vi "Begin.vi"() -> (1 "CameraDevRef":T1)   [LabVIEW 2011]
doc: "Called before other user functions, this VI is expected to open initial I/O refnums, load in file data, and do all program initialization. Notice that the <B>error out</B> terminal is simply used for data flow. Wiring it to other structures or subVIs ensures that this VI runs first."
uses:
  <vilib>/Rock Robotics/WPI/Camera/WPI_CameraDevRef.ctl
  <vilib>/Rock Robotics/SystemInterfaces/DIO/FPGA_DIOPWMChannel.ctl
  <vilib>/Rock Robotics/WPI/Joystick/WPI_JoystickDeviceEnum.ctl
  <vilib>/Rock Robotics/SystemInterfaces/AI/FPGA_AIChannel.ctl
  <vilib>/Rock Robotics/SystemInterfaces/DIO/FPGA_DIORelayChannel.ctl
  <vilib>/Rock Robotics/SystemInterfaces/DIO/FPGA_DIOChannel.ctl
  <vilib>/Rock Robotics/SystemInterfaces/AI/FPGA_AIGyroChannel.ctl
  <vilib>/Rock Robotics/WPI/Relay/WPI_RelayDirection.ctl
  <vilib>/Rock Robotics/WPI/MotorControl/WPI_MotorControlOpen Victor.vi
  <vilib>/Rock Robotics/WPI/MotorControl/WPI_MotorControlOpen Jaguar.vi
  Robot Global Data.vi
  <vilib>/Utility/file.llb/Read From Spreadsheet File (DBL).vi
  <vilib>/Rock Robotics/SystemInterfaces/Typedef/FPGA_TypedefDigitalModule.ctl
  <vilib>/Rock Robotics/WPI/Counter/WPI_CounterDigitalInputToDigitalSource.vi
  <vilib>/Rock Robotics/WPI/Encoder/WPI_EncoderType.ctl
  <vilib>/Rock Robotics/SystemInterfaces/Typedef/FPGA_TypedefAnalogModule.ctl
panel:
  out "Path and file":string
  in  "Balls In Robot At Start":dbl
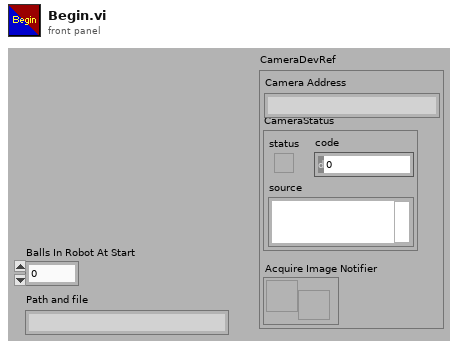
[diagram p1: front panel]
types:
  T1 = typedef "WPI_CameraDevRef.ctl" = cluster{"Camera Address":string, "CameraStatus":errorcluster, "Acquire Image Notifier":refnum<notifier>}
  T2 = typedef "FPGA_DIORelayChannel.ctl" = enum8{"Relay 1", "Relay 2", "Relay 3", "Relay 4", "Relay 5", "Relay 6", "Relay 7", "Relay 8", "Invalid"}
  T3 = typedef "WPI_RelayDirection.ctl" = enum16{"Both directions", "Forward only", "Reverse only"}
  T4 = typedef "FPGA_AIGyroChannel.ctl" = enum8{"AI 1", "AI 2", "Invalid"}
  T5 = typedef "FPGA_DIOChannel.ctl" = enum8{"DIO 1", "DIO 2", "DIO 3", "DIO 4", "DIO 5", "DIO 6", "DIO 7", "DIO 8", "DIO 9", "DIO 10", "DIO 11", "DIO 12", "DIO 13", "DIO 14", "Invalid"}
  T6 = typedef "FPGA_DIOPWMChannel.ctl" = enum8{"PWM 1", "PWM 2", "PWM 3", "PWM 4", "PWM 5", "PWM 6", "PWM 7", "PWM 8", "PWM 9", "PWM 10", "Invalid"}
  T7 = typedef "FPGA_AIChannel.ctl" = enum8{"AI 1", "AI 2", "AI 3", "AI 4", "AI 5", "AI 6", "AI 7", "AI 8", "Invalid"}
  T8 = typedef "WPI_JoystickDeviceEnum.ctl" = enum16{"USB 1", "USB 2", "USB 3", "USB 4", "Kinect 1", "Kinect 2"}
  T9 = typedef "WPI_CameraImageSize.ctl" = enum16{"640x480", "320x240", "160x120"}
  T10 = cluster{"fps":i32, "compression":i32, "Image Size":T9}
  T11 = typedef "WPI_MotorControlDeviceRef.ctl" = cluster{"DeviceStatus":errorcluster, "Type":enum16{"PWM", "CAN"}, "PWM":cluster{"Digital Module":T12, "PWM Channel":T6, "DeadBand":T13}, "CAN":cluster{"Device Number":u8, "Control Mode":T14, "Semaphore":T15, "Max Vout":dbl}, "Invert":bool, "TransformRef":T16, "InvTransformRef":T16}
  T12 = typedef "FPGA_TypedefDigitalModule.ctl" = enum16{"Digital Module 1", "Digital Module 2"}
  T13 = typedef "WPI_PWMDeadband.ctl" = cluster{"Name":string, "maxPositivePwm":i32, "minPositivePwm":i32, "centerPwm":i32, "maxNegativePwm":i32, "minNegativePwm":i32, "angularRange":u16}
  T14 = typedef "WPI_CANJaguar_ControlMode.ctl" = enum8{"Percent VBus", "Current", "Speed", "Position", "Voltage"}
  T15 = typedef "Semaphore RefNum" = refnum<k1>
  T16 = typedef "WPI_PWMTransform_ConPane.ctl" = refnum<vi>
  T17 = typedef "WPI_AnalogChannelDevRef.ctl" = cluster{"DevStatus":errorcluster, "Analog Module":T18, "Analog Channel":T7}
  T18 = typedef "FPGA_TypedefAnalogModule.ctl" = enum16{"Analog Module 1", "Analog Module 2"}
  T19 = typedef "WPI_ServoDeviceRef.ctl" = cluster{"DeviceStatus":errorcluster, "Digital Module":T12, "PWM Channel":T6, "DeadBand":T13}
  T20 = typedef "WPI_CameraWhite Balance Values.ctl" = enum16{"Auto", "Fixed indoor", "Fixed outdoor 1", "Fixed outdoor 2", "Fixed fluorescent 1", "Fixed fluorescent 2", "Hold current"}
  T21 = typedef "WPI_JoystickDevRef.ctl" = cluster{"Device":T8}
  T22 = typedef "WPI_RelayDevRef.ctl" = cluster{"DevStatus":errorcluster, "Relay Channel":T2, "Digital Module":T12, "Relay Direction":T3}
  T23 = typedef "WPI_CameraExposure Values.ctl" = enum16{"Auto", "Flicker-free 50 Hz", "Flicker-free 60 Hz", "Hold current"}
  T24 = typedef "WPI_EncoderType.ctl" = enum16{"1x", "2x", "4x"}
  T25 = typedef "WPI_DigitalInputDevRef.ctl" = cluster{"DevStatus":errorcluster, "DIO Channel":T5, "Digital Module":T12}
  T26 = typedef "FPGA_CounterEncoderSourceConvertionLVSourceType.ctl" = cluster{"DevStatus":errorcluster, "AnalogTriggerMode?":bool, "DigitalMode":cluster{"Digital Module":T12, "DIO Channel":T27}, "AnalogTriggerMode":cluster{"AnalogTriggerIndex":T28, "OutputType":T29}}
  T27 = typedef "FPGA_DIODigitalSourceChannel.ctl" = enum8{"DIO 1", "DIO 2", "DIO 3", "DIO 4", "DIO 5", "DIO 6", "DIO 7", "DIO 8", "DIO 9", "DIO 10", "DIO 11", "DIO 12", "DIO 13", "DIO 14", "Disabled"}
  T28 = typedef "FPGA_AnalogTriggerIndex.ctl" = enum8{"Trig 0", "Trig 1", "Trig 2", "Trig 3", "Trig 4", "Trig 5", "Trig 6", "Trig 7", "Invalid"}
  T29 = typedef "FPGA_AnalogTriggerOutType.ctl" = enum16{"InWindow", "TriggerState", "Rising", "Falling"}
  T30 = typedef "WPI_EncoderDevRef.ctl" = cluster{"DevStatus":errorcluster, "EncoderIndex":T31, "CounterIndex":T32, "DistancePerCount":dbl, "Decoding Type":T24}
  T31 = typedef "FPGA_EncoderIdx.ctl" = enum8{"Enc 0", "Enc 1", "Enc 2", "Enc 3", "Invalid"}
  T32 = typedef "FPGA_CounterCtrSystemIndex.ctl" = enum8{"Ctr 0", "Ctr 1", "Ctr 2", "Ctr 3", "Ctr 4", "Ctr 5", "Ctr 6", "Ctr 7", "Invalid"}
  T33 = typedef "WPI_GyroDevRef.ctl" = cluster{"DevStatus":errorcluster, "Analog Module":T18, "Analog Channel":T7, "Offset":dbl, "Gain (VoltsPerDegree/Second)":dbl}
  T34 = typedef "WPI_UltrasonicDeviceRef.ctl" = cluster{"DevStatus":errorcluster, "Ping Digital Module":T12, "Echo Digital Module":T12, "Ping Channel":T5, "Echo Channel":T5, "CntIndex":T32}
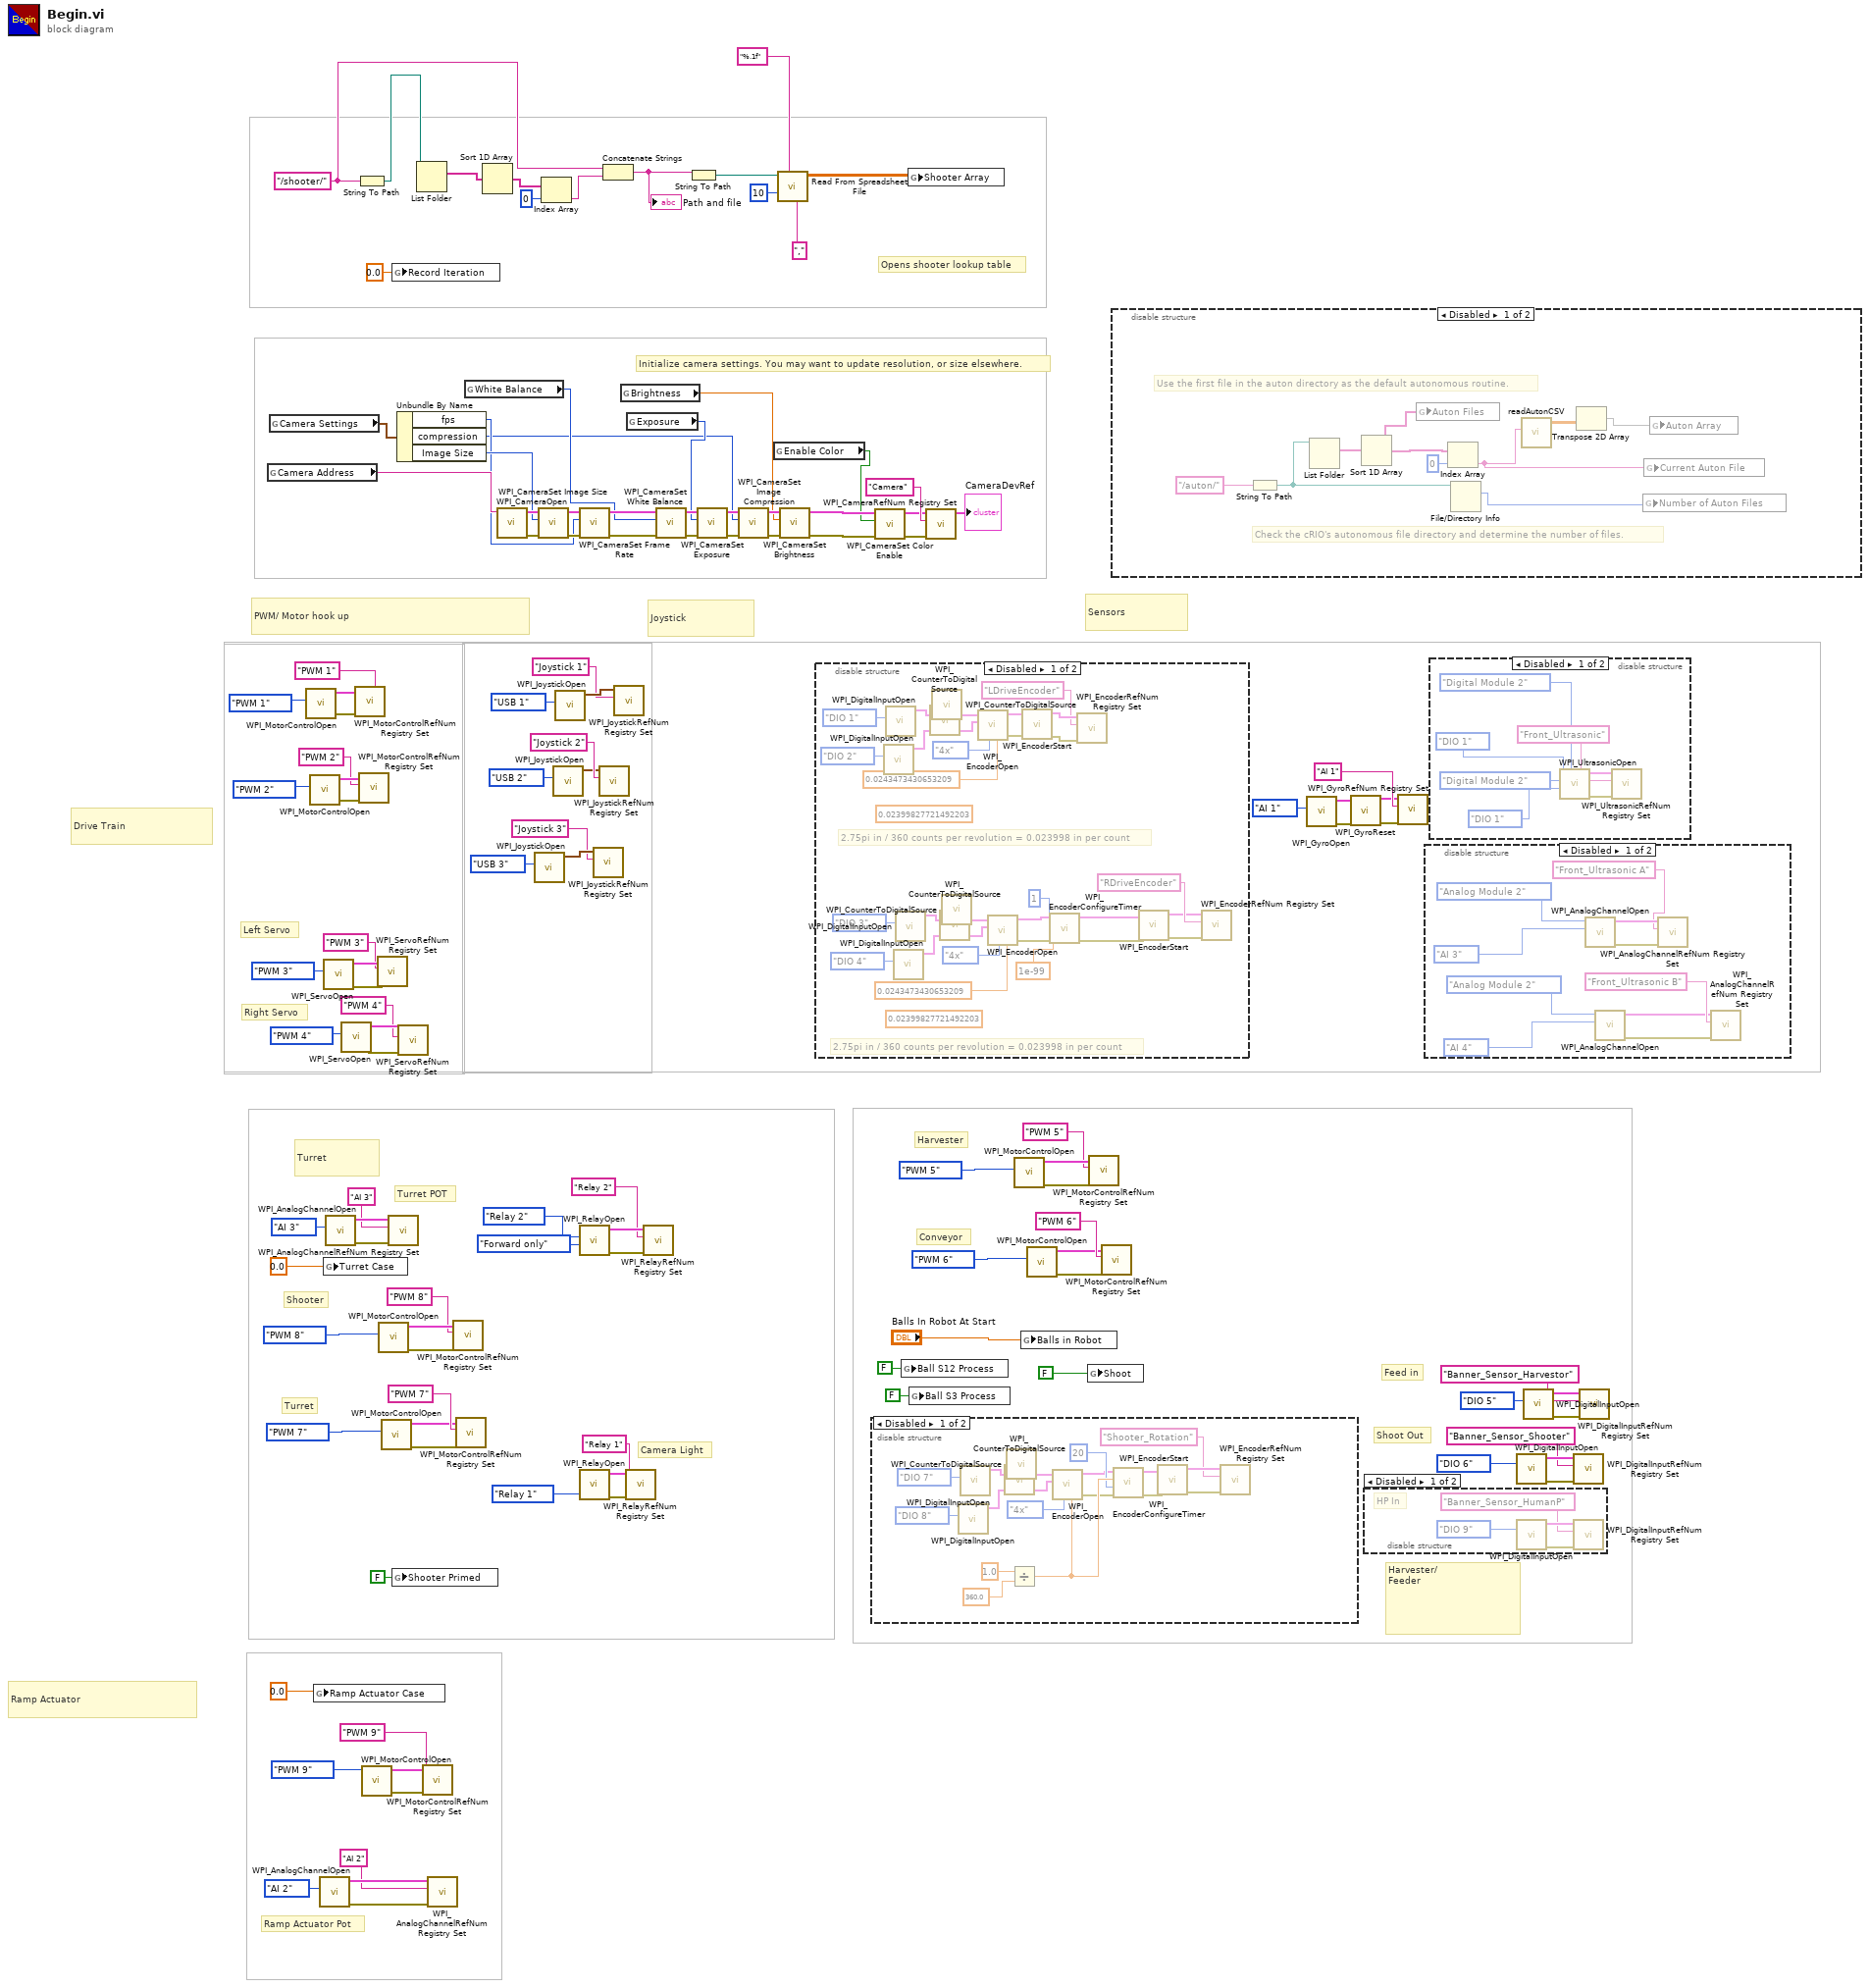
[diagram p0: block diagram]
diagram:
  w10 = "/shooter/" ("string")
  # "Opens shooter lookup table"
  # "Shoot Out"
  # "Feed in"
  # "Harvester"
  # "Conveyor"
  # "Shooter"
  # "Initialize camera settings. You may want to update resolution, or size elsewhere."
  # "Camera Light"
  # "Ramp Actuator Pot"
  # "Turret POT"
  # "Turret"
  # "Right Servo"
  # "Left Servo"
  # "Harvester/\nFeeder"
  # "Turret"
  # "Ramp Actuator"
  # "Drive Train"
  # "Sensors"
  # "Joystick"
  # "PWM/ Motor hook up"
  n1 = global read "Robot Global Data.vi" "Camera Address"() -> (w63:string)
  n2 = global read "Robot Global Data.vi" "Camera Settings"() -> (w62:T10)
  n3 = call-poly <vilib>:"WPI_MotorControlOpen.vi"("PWM Channel"=FPGA_DIOPWMChannel."PWM 1") -> ("error out"=w104:errorcluster, "MotorControlDeviceRef"=w106:T11)  [unwired: 9 in]
  n4 = call-poly <vilib>:"WPI_MotorControlOpen.vi"("PWM Channel"=FPGA_DIOPWMChannel."PWM 2") -> ("error out"=w102:errorcluster, "MotorControlDeviceRef"=w100:T11)  [unwired: 9 in]
  n5 = global write "Robot Global Data.vi" "Ramp Actuator Case"(0.0 ("Ramp Actuator Case")) -> ()
  n6 = call <vilib>:"WPI_AnalogChannelOpen.vi"("Analog Channel"=FPGA_AIChannel."AI 2") -> ("error out"=w88:errorcluster, "AIDeviceRef"=w89:T17)  [unwired: 9 in]
  n7 = call <vilib>:"WPI_ServoOpen.vi"("PWM Channel"=FPGA_DIOPWMChannel."PWM 3") -> ("error out"=w117:errorcluster, "ServoDeviceRef"=w122:T19)  [unwired: 9 in]
  n8 = global write "Robot Global Data.vi" "Turret Case"(0.0 ("Return To Home Case")) -> ()
  n9 = call <vilib>:"WPI_AnalogChannelOpen.vi"("Analog Channel"=FPGA_AIChannel."AI 3") -> ("error out"=w93:errorcluster, "AIDeviceRef"=w94:T17)  [unwired: 9 in]
  n10 = call <vilib>:"WPI_ServoOpen.vi"("PWM Channel"=FPGA_DIOPWMChannel."PWM 4") -> ("error out"=w116:errorcluster, "ServoDeviceRef"=w120:T19)  [unwired: 9 in]
  n11 = call <vilib>:"WPI_MotorControlRefNum Registry Set.vi"("error in (no error)"=w104, "refnum name"="PWM 1", "MotorControlDevRef"=w106) -> ()  [unwired: 7 in, 2 out]
  n12 = String To Path(string=w10) -> (path=w19:path)
  n13 = call <vilib>:"WPI_MotorControlRefNum Registry Set.vi"("error in (no error)"=w102, "refnum name"="PWM 2", "MotorControlDevRef"=w100) -> ()  [unwired: 7 in, 2 out]
  n14 = call-poly <vilib>:"WPI_MotorControlOpen.vi"("PWM Channel"=FPGA_DIOPWMChannel."PWM 9") -> ("error out"=w83:errorcluster, "MotorControlDeviceRef"=w84:T11)  [unwired: 9 in]
  n15 = call <vilib>:"WPI_ServoRefNum Registry Set.vi"("error in (no error)"=w117, "refnum name"="PWM 3", "ServoDeviceRef"=w122) -> ()  [unwired: 7 in, 2 out]
  n16 = call-poly <vilib>:"WPI_MotorControlOpen.vi"("PWM Channel"=FPGA_DIOPWMChannel."PWM 8") -> ("error out"=w46:errorcluster, "MotorControlDeviceRef"=w48:T11)  [unwired: 9 in]
  n17 = call-poly <vilib>:"WPI_MotorControlOpen.vi"("PWM Channel"=FPGA_DIOPWMChannel."PWM 7") -> ("error out"=w98:errorcluster, "MotorControlDeviceRef"=w96:T11)  [unwired: 9 in]
  n18 = call <vilib>:"WPI_AnalogChannelRefNum Registry Set.vi"("error in (no error)"=w93, "refnum name"="AI 3", "AIDeviceRef"=w94) -> ()  [unwired: 7 in, 2 out]
  n19 = global write "Robot Global Data.vi" "Record Iteration"(0.0 ("Record Iteration")) -> ()
  n20 = global write "Robot Global Data.vi" "Shooter Primed"(FALSE ("Ball S3 Process")) -> ()
  n21 = Unbundle By Name(w62) -> ("fps"=w60:i32, "compression"=w57:i32, "Image Size"=w61:T9)
  n22 = call <vilib>:"WPI_ServoRefNum Registry Set.vi"("error in (no error)"=w116, "refnum name"="PWM 4", "ServoDeviceRef"=w120) -> ()  [unwired: 7 in, 2 out]
  n23 = List Folder(path=w19) -> (filenames=w18:string[])  [unwired: 1 in, 5 out]
  n24 = call <vilib>:"WPI_MotorControlRefNum Registry Set.vi"("error in (no error)"=w83, "refnum name"="PWM 9", "MotorControlDevRef"=w84) -> ()  [unwired: 7 in, 2 out]
  n25 = call <vilib>:"WPI_AnalogChannelRefNum Registry Set.vi"("error in (no error)"=w88, "refnum name"="AI 2", "AIDeviceRef"=w89) -> ()  [unwired: 7 in, 2 out]
  n26 = call <vilib>:"WPI_MotorControlRefNum Registry Set.vi"("error in (no error)"=w46, "refnum name"="PWM 8", "MotorControlDevRef"=w48) -> ()  [unwired: 7 in, 2 out]
  n27 = call <vilib>:"WPI_MotorControlRefNum Registry Set.vi"("error in (no error)"=w98, "refnum name"="PWM 7", "MotorControlDevRef"=w96) -> ()  [unwired: 7 in, 2 out]
  n28 = global read "Robot Global Data.vi" "White Balance"() -> (w59:T20)
  n29 = Sort 1D Array(array=w18) -> (sorted array=w17:string[])
  n30 = call <vilib>:"WPI_CameraOpen.vi"("Camera Address"=w63) -> ("error out"=w69:errorcluster, "CameraDevRef"=w70:T1)  [unwired: 1 in, 8 out]
  n31 = call <vilib>:"WPI_JoystickOpen.vi"("JoystickDevice"=WPI_JoystickDeviceEnum."USB 3") -> ("JoystickDevRef"=w109:T21)  [unwired: 10 in]
  n32 = call <vilib>:"WPI_CameraSet Image Size.vi"("error in (no error)"=w69, "Image Size"=w61, "CameraDevRef"=w70) -> ("error out"=w68:errorcluster, "CameraDevRef Out"=w71:T1)  [unwired: 7 out]
  n33 = Index Array(array=w17, index=0) -> (element=w9:string)
  n34 = call <vilib>:"WPI_JoystickOpen.vi"("JoystickDevice"=WPI_JoystickDeviceEnum."USB 2") -> ("JoystickDevRef"=w112:T21)  [unwired: 10 in]
  n35 = call <vilib>:"WPI_JoystickOpen.vi"("JoystickDevice"=WPI_JoystickDeviceEnum."USB 1") -> ("JoystickDevRef"=w115:T21)  [unwired: 10 in]
  n36 = call <vilib>:"WPI_CameraSet Frame Rate.vi"("error in (no error)"=w68, "Frame Rate (fps)"=w60, "CameraDevRef"=w71) -> ("error out"=w67:errorcluster, "CameraDevRef Out"=w73:T1)  [unwired: 7 out]
  n37 = call <vilib>:"WPI_RelayOpen.vi"("Relay Direction"=WPI_RelayDirection."Forward only", "Relay Channel"=FPGA_DIORelayChannel."Relay 2") -> ("error out"=w4:errorcluster, "RelayDevRef"=w5:T22)  [unwired: 8 in]
  n38 = call <vilib>:"WPI_RelayOpen.vi"("Relay Channel"=FPGA_DIORelayChannel."Relay 1") -> ("error out"=w80:errorcluster, "RelayDevRef"=w79:T22)  [unwired: 9 in]
  n39 = call <vilib>:"WPI_JoystickRefNum Registry Set.vi"("refnum name"="Joystick 3", "JoystickDevRef"=w109) -> ()  [unwired: 8 in, 2 out]
  n40 = call <vilib>:"WPI_JoystickRefNum Registry Set.vi"("refnum name"="Joystick 2", "JoystickDevRef"=w112) -> ()  [unwired: 8 in, 2 out]
  n41 = Concatenate Strings(w10, w9) -> (w12:string)
  "Path and file" <- w12
  n42 = call <vilib>:"WPI_JoystickRefNum Registry Set.vi"("refnum name"="Joystick 1", "JoystickDevRef"=w115) -> ()  [unwired: 8 in, 2 out]
  n43 = global read "Robot Global Data.vi" "Brightness"() -> (w56:dbl)
  n44 = call <vilib>:"WPI_RelayRefNum Registry Set.vi"("error in (no error)"=w80, "refnum name"="Relay 1", "RelayDevRef"=w79) -> ()  [unwired: 7 in, 2 out]
  n45 = global read "Robot Global Data.vi" "Exposure"() -> (w58:T23)
  n46 = call <vilib>:"WPI_RelayRefNum Registry Set.vi"("error in (no error)"=w4, "refnum name"="Relay 2", "RelayDevRef"=w5) -> ()  [unwired: 7 in, 2 out]
  n47 = call <vilib>:"WPI_CameraSet White Balance.vi"("error in (no error)"=w67, "White Balance"=w59, "CameraDevRef"=w73) -> ("error out"=w66:errorcluster, "CameraDevRef Out"=w72:T1)  [unwired: 7 out]
  n48 = String To Path(string=w12) -> (path=w11:path)
  n49 = call <vilib>:"WPI_CameraSet Exposure.vi"("error in (no error)"=w66, "Exposure"=w58, "CameraDevRef"=w72) -> ("error out"=w65:errorcluster, "CameraDevRef Out"=w75:T1)  [unwired: 7 out]
  n50 = call <vilib>:"WPI_CameraSet Image Compression.vi"("error in (no error)"=w65, "Compression"=w57, "CameraDevRef"=w75) -> ("error out"=w64:errorcluster, "CameraDevRef Out"=w74:T1)  [unwired: 7 out]
  n51 = global read "Robot Global Data.vi" "Enable Color"() -> (w51:bool)
  n52 = call-poly <vilib>:"Read From Spreadsheet File.vi"("delimiter (\\t)"="," ("delimiter (\\t)"), "format (%.3f)"="%.1f", "number of rows (all:-1)"=10, "file path (dialog if empty)"=w11) -> ("all rows"=w8:dbl[][])  [unwired: 1 in, 6 out]
  n53 = call <vilib>:"WPI_CameraSet Brightness.vi"("error in (no error)"=w64, "Brightness"=w56, "CameraDevRef"=w74) -> ("error out"=w54:errorcluster, "CameraDevRef Out"=w55:T1)  [unwired: 7 out]
  n54 = disable-structure shown="Disabled" {
    frame Disabled {
      (unwired) 0.02399827721492203 ("DistancePerCount")
      (unwired) 0.02399827721492203 ("DistancePerCount")
      # "2.75pi in / 360 counts per revolution = 0.023998 in per count"
      # "2.75pi in / 360 counts per revolution = 0.023998 in per count"
      n55 = call <vilib>:"WPI_DigitalInputOpen.vi"("DIO Channel"=FPGA_DIOChannel."DIO 2") -> ("DigitalInputDevRef"=w147:T25)  [unwired: 9 in, 1 out]
      n56 = call <vilib>:"WPI_DigitalInputOpen.vi"("DIO Channel"=FPGA_DIOChannel."DIO 1") -> ("DigitalInputDevRef"=w144:T25)  [unwired: 9 in, 1 out]
      n57 = call <vilib>:"WPI_DigitalInputOpen.vi"("DIO Channel"=FPGA_DIOChannel."DIO 4") -> ("DigitalInputDevRef"=w138:T25)  [unwired: 9 in, 1 out]
      n58 = call <vilib>:"WPI_DigitalInputOpen.vi"("DIO Channel"=FPGA_DIOChannel."DIO 3") -> ("DigitalInputDevRef"=w141:T25)  [unwired: 9 in, 1 out]
      n59 = call-poly <vilib>:"WPI_CounterToDigitalSource.vi"("DigitalInputDevRef"=w147) -> ("Digital Source"=w148:T26)  [unwired: 6 in]
      n60 = call-poly <vilib>:"WPI_CounterToDigitalSource.vi"("DigitalInputDevRef"=w144) -> ("Digital Source"=w143:T26)  [unwired: 6 in]
      n61 = call-poly <vilib>:"WPI_CounterToDigitalSource.vi"("DigitalInputDevRef"=w138) -> ("Digital Source"=w137:T26)  [unwired: 6 in]
      n62 = call-poly <vilib>:"WPI_CounterToDigitalSource.vi"("DigitalInputDevRef"=w141) -> ("Digital Source"=w142:T26)  [unwired: 6 in]
      n63 = call <vilib>:"WPI_EncoderOpen.vi"("DistancePerCount"=0.0243473430653209, "Decoding Type"=WPI_EncoderType."4x", "BSource"=w148, "ASource"=w143) -> ("error out"=w150:errorcluster, "EncoderDevRef"=w151:T30)  [unwired: 6 in]
      n64 = call <vilib>:"WPI_EncoderOpen.vi"("DistancePerCount"=0.0243473430653209, "Decoding Type"=WPI_EncoderType."4x", "BSource"=w137, "ASource"=w142) -> ("error out"=w134:errorcluster, "EncoderDevRef"=w133:T30)  [unwired: 6 in]
      n65 = call <vilib>:"WPI_EncoderStart.vi"("error in (no error)"=w150, "EncoderDevRef"=w151) -> ("error out"=w153:errorcluster, "EncoderDevRef"=w152:T30)  [unwired: 8 in]
      n66 = call <vilib>:"WPI_EncoderConfigureTimer.vi"("error in (no error)"=w134, "Number Samples to Average"=u8 1, "Minimum Rate"=1e-99, "EncoderDevRef"=w133) -> ("error out"=w129:errorcluster, "EncoderDevRef"=w130:T30)  [unwired: 6 in]
      n67 = call <vilib>:"WPI_EncoderRefNum Registry Set.vi"("error in (no error)"=w153, "refnum name"="LDriveEncoder", "EncoderDevRef"=w152) -> ()  [unwired: 7 in, 2 out]
      n68 = call <vilib>:"WPI_EncoderStart.vi"("error in (no error)"=w129, "EncoderDevRef"=w130) -> ("error out"=w127:errorcluster, "EncoderDevRef"=w128:T30)  [unwired: 8 in]
      n69 = call <vilib>:"WPI_EncoderRefNum Registry Set.vi"("error in (no error)"=w127, "refnum name"="RDriveEncoder", "EncoderDevRef"=w128) -> ()  [unwired: 7 in, 2 out]
    }
    frame Enabled {
    }
  }
  n70 = disable-structure shown="Disabled" {
    frame Disabled {
      n71 = call <vilib>:"WPI_DigitalInputOpen.vi"("DIO Channel"=FPGA_DIOChannel."DIO 8") -> ("DigitalInputDevRef"=w158:T25)  [unwired: 9 in, 1 out]
      n72 = call <vilib>:"WPI_DigitalInputOpen.vi"("DIO Channel"=FPGA_DIOChannel."DIO 7") -> ("DigitalInputDevRef"=w155:T25)  [unwired: 9 in, 1 out]
      n73 = call-poly <vilib>:"WPI_CounterToDigitalSource.vi"("DigitalInputDevRef"=w158) -> ("Digital Source"=w159:T26)  [unwired: 6 in]
      n74 = call-poly <vilib>:"WPI_CounterToDigitalSource.vi"("DigitalInputDevRef"=w155) -> ("Digital Source"=w154:T26)  [unwired: 6 in]
      n75 = Divide(x=1.0, y=360.0) -> (x/y=w171:dbl)
      n76 = call <vilib>:"WPI_EncoderOpen.vi"("DistancePerCount"=w171, "Decoding Type"=WPI_EncoderType."4x", "BSource"=w159, "ASource"=w154) -> ("error out"=w162:errorcluster, "EncoderDevRef"=w163:T30)  [unwired: 6 in]
      n77 = call <vilib>:"WPI_EncoderConfigureTimer.vi"("error in (no error)"=w162, "Number Samples to Average"=u8 20, "Minimum Rate"=w171, "EncoderDevRef"=w163) -> ("error out"=w166:errorcluster, "EncoderDevRef"=w165:T30)  [unwired: 6 in]
      n78 = call <vilib>:"WPI_EncoderStart.vi"("error in (no error)"=w166, "EncoderDevRef"=w165) -> ("error out"=w168:errorcluster, "EncoderDevRef"=w167:T30)  [unwired: 8 in]
      n79 = call <vilib>:"WPI_EncoderRefNum Registry Set.vi"("error in (no error)"=w168, "refnum name"="Shooter_Rotation", "EncoderDevRef"=w167) -> ()  [unwired: 7 in, 2 out]
    }
    frame Enabled {
    }
  }
  n80 = call <vilib>:"WPI_CameraSet Color Enable.vi"("error in (no error)"=w54, "Color Enabled"=w51, "CameraDevRef"=w55) -> ("error out"=w52:errorcluster, "CameraDevRef Out"=w53:T1)  [unwired: 7 in]
  n81 = global write "Robot Global Data.vi" "Ball S12 Process"(FALSE ("Ball S12 Process")) -> ()
  n82 = global write "Robot Global Data.vi" "Shooter Array"(w8) -> ()
  n83 = global write "Robot Global Data.vi" "Ball S3 Process"(FALSE ("Ball S3 Process")) -> ()
  n84 = call <vilib>:"WPI_CameraRefNum Registry Set.vi"("error in (no error)"=w52, "refnum name"="Camera", "CameraDevRef"=w53) -> ("CameraDevRef"=→"CameraDevRef":T1)  [unwired: 8 out]
  n85 = call-poly <vilib>:"WPI_MotorControlOpen.vi"("PWM Channel"=FPGA_DIOPWMChannel."PWM 5") -> ("error out"=w42:errorcluster, "MotorControlDeviceRef"=w44:T11)  [unwired: 9 in]
  n86 = global write "Robot Global Data.vi" "Balls in Robot"("Balls In Robot At Start") -> ()
  n87 = call-poly <vilib>:"WPI_MotorControlOpen.vi"("PWM Channel"=FPGA_DIOPWMChannel."PWM 6") -> ("error out"=w41:errorcluster, "MotorControlDeviceRef"=w39:T11)  [unwired: 9 in]
  n88 = global write "Robot Global Data.vi" "Shoot"(FALSE ("Ball S12 Process")) -> ()
  n89 = call <vilib>:"WPI_MotorControlRefNum Registry Set.vi"("error in (no error)"=w42, "refnum name"="PWM 5", "MotorControlDevRef"=w44) -> ()  [unwired: 7 in, 2 out]
  n90 = call <vilib>:"WPI_MotorControlRefNum Registry Set.vi"("error in (no error)"=w41, "refnum name"="PWM 6", "MotorControlDevRef"=w39) -> ()  [unwired: 7 in, 2 out]
  n91 = disable-structure shown="Disabled" {
    frame Disabled {
      # "Check the cRIO's autonomous file directory and determine the number of files."
      # "Use the first file in the auton directory as the default autonomous routine."
      n92 = String To Path(string="/auton/") -> (path=w176:path)
      n93 = List Folder(path=w176) -> (filenames=w175:string[])  [unwired: 1 in, 5 out]
      n94 = Sort 1D Array(array=w175) -> (sorted array=w173:string[])
      n95 = global write "Robot Global Data.vi" "Auton Files"(w173) -> ()
      n96 = Index Array(array=w173, index=0) -> (element=w179:string)
      n97 = File/Directory Info(path=w176) -> (size=w180:i64)  [unwired: 1 in, 6 out]
      n98 = call "readAutonCSV.vi"("AutonFile"=w179) -> ("AutonArray"=w172:dbl[][])  [unwired: 7 in]
      n99 = Transpose 2D Array(2D array=w172) -> (transposed array=w178:dbl[][])
      n100 = global write "Robot Global Data.vi" "Number of Auton Files"(w180) -> ()
      n101 = global write "Robot Global Data.vi" "Current Auton File"(w179) -> ()
      n102 = global write "Robot Global Data.vi" "Auton Array"(w178) -> ()
    }
    frame Enabled {
    }
  }
  n103 = call <vilib>:"WPI_GyroOpen.vi"("Analog Channel"=FPGA_AIGyroChannel."AI 1") -> ("error out"=w22:errorcluster, "GyroDevRef"=w23:T33)  [unwired: 8 in, 1 out]
  n104 = call <vilib>:"WPI_GyroReset.vi"("error in (no error)"=w22, "GyroDevRef"=w23) -> ("error out"=w21:errorcluster, "GyroDevRef"=w20:T33)  [unwired: 8 in]
  n105 = disable-structure shown="Disabled" {
    frame Disabled {
      # "HP In"
      n106 = call <vilib>:"WPI_DigitalInputOpen.vi"("DIO Channel"=FPGA_DIOChannel."DIO 9") -> ("error out"=w183:errorcluster, "DigitalInputDevRef"=w182:T25)  [unwired: 9 in]
      n107 = call <vilib>:"WPI_DigitalInputRefNum Registry Set.vi"("error in (no error)"=w183, "refnum name"="Banner_Sensor_HumanP", "DigitalInputDevRef"=w182) -> ()  [unwired: 7 in, 2 out]
    }
    frame Enabled {
    }
  }
  n108 = call <vilib>:"WPI_GyroRefNum Registry Set.vi"("error in (no error)"=w21, "refnum name"="AI 1", "GyroDevRef"=w20) -> ()  [unwired: 7 in, 2 out]
  n109 = disable-structure shown="Disabled" {
    frame Disabled {
      n110 = call <vilib>:"WPI_AnalogChannelOpen.vi"("Analog Channel"=FPGA_AIChannel."AI 3", "Analog Module (Module 1)"=FPGA_TypedefAnalogModule."Analog Module 2") -> ("error out"=w190:errorcluster, "AIDeviceRef"=w189:T17)  [unwired: 8 in]
      n111 = call <vilib>:"WPI_AnalogChannelOpen.vi"("Analog Channel"=FPGA_AIChannel."AI 4", "Analog Module (Module 1)"=FPGA_TypedefAnalogModule."Analog Module 2") -> ("error out"=w185:errorcluster, "AIDeviceRef"=w186:T17)  [unwired: 8 in]
      n112 = call <vilib>:"WPI_AnalogChannelRefNum Registry Set.vi"("error in (no error)"=w190, "refnum name"="Front_Ultrasonic A", "AIDeviceRef"=w189) -> ()  [unwired: 7 in, 2 out]
      n113 = call <vilib>:"WPI_AnalogChannelRefNum Registry Set.vi"("error in (no error)"=w185, "refnum name"="Front_Ultrasonic B", "AIDeviceRef"=w186) -> ()  [unwired: 7 in, 2 out]
    }
    frame Enabled {
    }
  }
  n114 = disable-structure shown="Disabled" {
    frame Disabled {
      n115 = call <vilib>:"WPI_UltrasonicOpen.vi"("Ping Digital Module (Module 1)"=FPGA_TypedefDigitalModule."Digital Module 2", "Echo DIO Channel"=FPGA_DIOChannel."DIO 1", "Echo Digital Module (Module 1)"=FPGA_TypedefDigitalModule."Digital Module 2", "Ping DIO Channel"=FPGA_DIOChannel."DIO 1") -> ("error out"=w201:errorcluster, "UltrasonicDevRef"=w200:T34)  [unwired: 6 in]
      n116 = call <vilib>:"WPI_UltrasonicRefNum Registry Set.vi"("error in (no error)"=w201, "refnum name"="Front_Ultrasonic", "UltrasonicDevRef"=w200) -> ()  [unwired: 7 in, 2 out]
    }
    frame Enabled {
    }
  }
  n117 = call <vilib>:"WPI_DigitalInputOpen.vi"("DIO Channel"=FPGA_DIOChannel."DIO 6") -> ("error out"=w32:errorcluster, "DigitalInputDevRef"=w31:T25)  [unwired: 9 in]
  n118 = call <vilib>:"WPI_DigitalInputOpen.vi"("DIO Channel"=FPGA_DIOChannel."DIO 5") -> ("error out"=w35:errorcluster, "DigitalInputDevRef"=w34:T25)  [unwired: 9 in]
  n119 = call <vilib>:"WPI_DigitalInputRefNum Registry Set.vi"("error in (no error)"=w32, "refnum name"="Banner_Sensor_Shooter", "DigitalInputDevRef"=w31) -> ()  [unwired: 7 in, 2 out]
  n120 = call <vilib>:"WPI_DigitalInputRefNum Registry Set.vi"("error in (no error)"=w35, "refnum name"="Banner_Sensor_Harvestor", "DigitalInputDevRef"=w34) -> ()  [unwired: 7 in, 2 out]
